vi "ReHomeWinch.vi"(11 "Buttons":bool[](array[boolean])) -> ()   [LabVIEW 2015]
uses:
  <vilib>/Rock Robotics/WPI/CAN/TalonSRX/WPI_CANTalonSRX_APIControlMode.ctl
  <vilib>/Rock Robotics/WPI/CAN/TalonSRX/WPI_CANTalonSRX_APIFeedbackSelect.ctl
panel:
  in  "Winch PID Gains":T1={"proportional gain (Kc)"=10.0, "integral time (Ti, min)"=0.0, "derivative time (Td, min)"=4.0}
  in  "error in (no error)":errorcluster
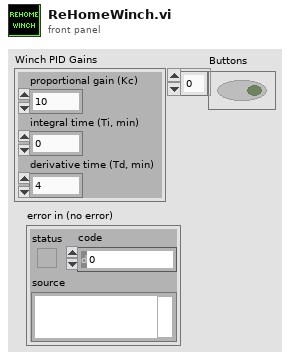
[diagram p1: front panel]
types:
  T1 = cluster{"proportional gain (Kc)":dbl, "integral time (Ti, min)":dbl, "derivative time (Td, min)":dbl}
  T2 = typedef "WPI_CANTalonSRX_APIControlMode.ctl" = enum8{"Percent VBus", "Speed", "Position", "Slave", "Unchanged / Invalid", "Voltage Compensation", "Current", "Motion Profile"}
  T3 = typedef "WPI_CANTalonSRX_APIFeedbackSelect.ctl" = enum16{"Digital Quadrature Encoder", "Analog Potentiometer", "Analog Encoder", "Count on Quad-A (Rising-Edge)", "Count on Quad-A (Falling-Edge)", "CTR Magnetic Enc (Absolute)", "CTR Magnetic Enc (Relative)", "Pulse Width"}
  T4 = typedef "WPI_MotorControlDeviceRef.ctl" = cluster{"DeviceStatus":errorcluster, "Type":T5, "PWM":cluster{"PWM Channel":T6, "DeadBand":T7}, "CAN":cluster{"Device Number":u8, "Control Mode":T8, "Semaphore":T9, "Max Vout":dbl, "TalonSRX Control Mode":T2}, "Invert":bool}
  T5 = typedef "WPI_MotorControlType.ctl" = enum16{"PWM", "CAN", "CANTalonSRX"}
  T6 = typedef "FPGA_DIOPWMChannel.ctl" = enum8{"PWM 0", "PWM 1", "PWM 2", "PWM 3", "PWM 4", "PWM 5", "PWM 6", "PWM 7", "PWM 8", "PWM 9", "PWM MXP 0", "PWM MXP 1", "PWM MXP 2", "PWM MXP 3", "PWM MXP 4", "PWM MXP 5", "PWM MXP 6", "PWM MXP 7", "PWM MXP 8", "PWM MXP 9", "Invalid"}
  T7 = typedef "WPI_PWMDeadband.ctl" = cluster{"Name":string, "maxPositivePwm":i32, "minPositivePwm":i32, "centerPwm":i32, "maxNegativePwm":i32, "minNegativePwm":i32, "angularRange":u16}
  T8 = typedef "WPI_CANJaguar_ControlMode.ctl" = enum8{"Percent VBus", "Current", "Speed", "Position", "Voltage"}
  T9 = typedef "Semaphore RefNum" = refnum<k1>
  T10 = typedef "WPI_SwitchDevRef.ctl" = cluster{"DevStatus":errorcluster, "DIO Channel":T11, "CntIndex":T12, "Normally Closed":bool}
  T11 = typedef "FPGA_DIOChannel.ctl" = enum8{"DIO 0", "DIO 1", "DIO 2", "DIO 3", "DIO 4", "DIO 5", "DIO 6", "DIO 7", "DIO 8", "DIO 9", "DIO MXP 0", "DIO MXP 1", "DIO MXP 2", "DIO MXP 3", "DIO MXP 4", "DIO MXP 5", "DIO MXP 6", "DIO MXP 7", "DIO MXP 8", "DIO MXP 9", "DIO MXP 10", "DIO MXP 11", "DIO MXP 12", "DIO MXP 13", "DIO MXP 14", "DIO MXP 15", "Invalid"}
  T12 = typedef "FPGA_CounterCtrSystemIndex.ctl" = enum8{"Ctr 0", "Ctr 1", "Ctr 2", "Ctr 3", "Ctr 4", "Ctr 5", "Ctr 6", "Ctr 7", "Invalid"}
  T13 = typedef "WPI_CANTalonSRX_GlobalStatus.ctl" = cluster{"Applied Throttle":dbl, "Module Enabled":bool, "CAN Error":errorcluster, "Closed Loop Error":dbl, "Forward Limit Switch Closed":bool, "Reverse Limit Switch Closed":bool, "Sensor Position":dbl, "Sensor Velocity":dbl, "Current":dbl, "Sticky Fault - Over Temp":bool, "Sticky Fault - Under Voltage":bool, "Sticky Fault - Forward Limit":bool, "Sticky Fault - Reverse Limit":bool, "Sticky Fault - Forward Soft Limit":bool, "Sticky Fault - Reverse Soft Limit":bool, "Brake is Enabled":bool, "Encoder Position":dbl, "Encoder Velocity":dbl, "Encoder Index Count":dbl, "Encoder A Pin State":bool, "Encoder B Pin State":bool, "Encoder Index Pin State":bool, "Analog In":dbl, "Analog In Velocity":dbl, "Temperature (C)":dbl, "Battery Voltage":dbl, "Control 5 Is Supported":bool, "Current Profile Slot Select":dbl, "Pos Div 8":bool, "Vel Div 4":bool, "Pulse Width Position":i32, "Pulse Width Velocity":i32, "Pulse Width Rise To Rise (us)":i32, "Pulse Width Rise To Fall (us)":i32, "Mot Prof Active Is Under Run":bool, "Mot Prof Active Has Under Run":bool, "Mot Prof Active Is Last":bool, "Mot Prof Active Velocity Only":bool, "Mot Prof Active Is Valid":bool, "Mot Prof Buffer Is Full":bool, "Mot Prof Active Profile Slot Select":i32, "Mot Prof NextID":i32, "Mot Prof Count":i32, "Mot Prof Active Velocity":dbl, "Mot Prof Active Position":dbl, "Mot Prof Output Enable":i32}
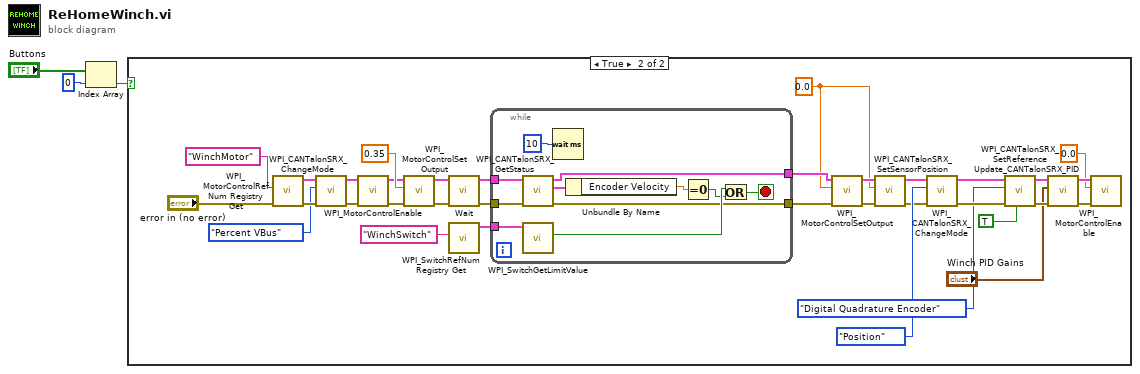
[diagram p0: block diagram]
diagram:
  n1 = Index Array(array="Buttons", index=0) -> (element=w1:bool)
  n2 = case shown="True" w1 {
    frame False {
    }
    frame True {
      w6 = 0.0 ("Output")
      n3 = call <vilib>:"WPI_MotorControlRefNum Registry Get.vi"("error in (no error)"="error in (no error)", "refnum name"="WinchMotor") -> ("error out"=w15:errorcluster, "MotorControlDevRef"=w16:T4)  [unwired: 8 in]
      n4 = call <vilib>:"WPI_CANTalonSRX_ChangeMode.vi"("error in (no error)"=w15, "Control Mode"=WPI_CANTalonSRX_APIControlMode."Percent VBus", "CAN Talon SRX Ref"=w16) -> ("error out"=w11:errorcluster, "CAN Talon SRX Ref"=w12:T4)  [unwired: 7 in]
      n5 = call <vilib>:"WPI_MotorControlEnable.vi"("error in (no error)"=w11, "CAN MotorDevRef"=w12) -> ("error out"=w9:errorcluster, "CAN MotorDevRef"=w10:T4)  [unwired: 8 in]
      n6 = call <vilib>:"WPI_MotorControlSetOutput.vi"("error in (no error)"=w9, "Output"=0.35, "MotorControlDevRef"=w10) -> ("error out"=w19:errorcluster, "MotorControlDevRef"=w20:T4)  [unwired: 6 in, 1 out]
      n7 = call "Wait.vi"("error in (no error)"=w19, "MotorControlDeviceRefIn"=w20) -> ("error out"=w17:errorcluster, "MotorControlDeviceRefOut"=w18:T4)  [unwired: 8 in]
      n8 = call <vilib>:"WPI_SwitchRefNum Registry Get.vi"("refnum name"="WinchSwitch") -> ("SwitchDevRef"=w22:T10)  [unwired: 9 in, 1 out]
      n9 = while {
        tunnel: [w41] -> w34
        tunnel: [w40] -> w35
        tunnel: w22 -> [w48]
        tunnel: w18 -> [w39]
        tunnel: w17 -> [w38]
        stop <- w43 stop-if-true
        n10 = call <vilib>:"WPI_CANTalonSRX_GetStatus.vi"("error in (no error)"=w38, "CAN Talon SRX Ref"=w39) -> ("error out"=w40:errorcluster, "Talon SRX Status"=w46:T13, "CAN Talon SRX Ref"=w41:T4)  [unwired: 7 in]
        n11 = call <vilib>:"WPI_SwitchGetLimitValue.vi"("SwitchDevRef"=w48) -> ("Switch Pressed"=w47:bool)  [unwired: 8 in, 2 out]
        n12 = Wait (ms)(milliseconds to wait=u32 10) -> ()  [unwired: 1 out]
        n13 = Unbundle By Name(w46) -> ("Encoder Velocity"=w45:dbl)
        n14 = Equal To 0?(x=w45) -> (x = 0?=w42:bool)
        n15 = Or(x=w47, y=w42) -> (x .or. y?=w43:bool)
      }
      n16 = call <vilib>:"WPI_MotorControlSetOutput.vi"("error in (no error)"=w35, "Output"=w6, "MotorControlDevRef"=w34) -> ("error out"=w8:errorcluster, "MotorControlDevRef"=w7:T4)  [unwired: 6 in, 1 out]
      n17 = call <vilib>:"WPI_CANTalonSRX_SetSensorPosition.vi"("error in (no error)"=w8, "New Sensor Position"=w6, "CAN Talon SRX Ref"=w7) -> ("error out"=w4:errorcluster, "CAN Talon SRX Ref"=w5:T4)  [unwired: 7 in]
      n18 = call <vilib>:"WPI_CANTalonSRX_ChangeMode.vi"("error in (no error)"=w4, "Control Mode"=WPI_CANTalonSRX_APIControlMode."Position", "CAN Talon SRX Ref"=w5) -> ("error out"=w31:errorcluster, "CAN Talon SRX Ref"=w32:T4)  [unwired: 7 in]
      n19 = call <vilib>:"WPI_CANTalonSRX_SetReference.vi"("Reverse Closed-Loop Output"=TRUE, "error in (no error)"=w31, "Feedback Reference"=WPI_CANTalonSRX_APIFeedbackSelect."Digital Quadrature Encoder", "CAN Talon SRX Ref"=w32) -> ("error out"=w29:errorcluster, "CAN Talon SRX Ref"=w28:T4)  [unwired: 6 in]
      n20 = call "Update_CANTalonSRX_PID.vi"("error in (no error)"=w29, "PID Gains"="Winch PID Gains", "CAN Talon SRX Ref"=w28) -> ("error out"=w26:errorcluster, "CAN Talon SRX Ref Out"=w25:T4)  [unwired: 7 in]
      n21 = call <vilib>:"WPI_MotorControlEnable.vi"("error in (no error)"=w26, "Encoder Initial Position"=0.0, "CAN MotorDevRef"=w25) -> ()  [unwired: 7 in, 2 out]
    }
  }
